vi "例7.4利用XY图显示单条曲线.vi"() -> ()   [LabVIEW 2017]
panel:
  out "XY图 2":cluster{"X":dbl, "Y":dbl}[](graph)
  out "XY图":cluster{dbl[], dbl[]}(graph)
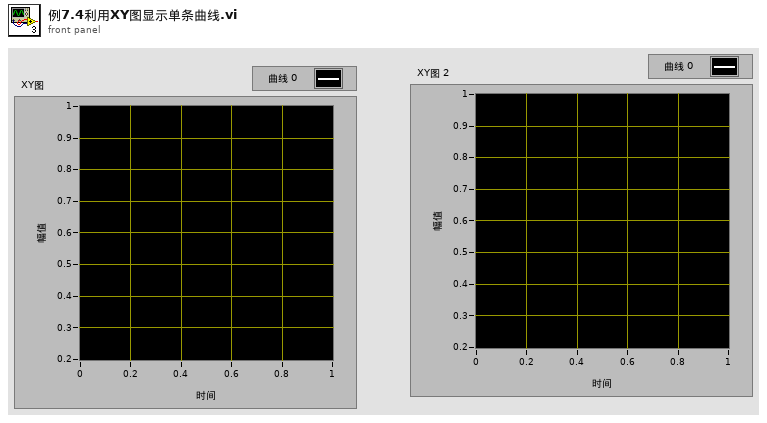
[diagram p1: front panel]
types:
  T1 = cluster{"number: 0 to 1":dbl, "number: 0 to 1":dbl}
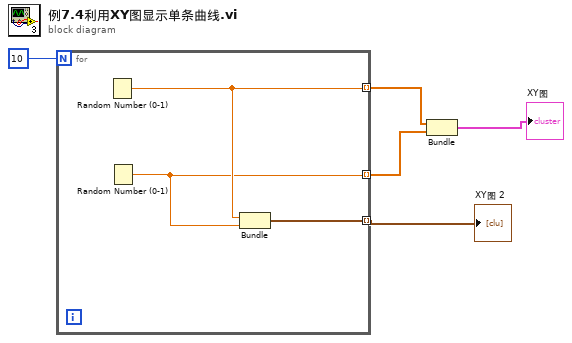
[diagram p0: block diagram]
diagram:
  n1 = for {
    N: 10 -> [_]
    tunnel: [w8] -> w4 mode=indexing
    tunnel: [w7] -> w3 mode=indexing
    tunnel: [w6] -> w1 mode=indexing
    n2 = Random Number (0-1)() -> (number: 0 to 1=w8:dbl)
    n3 = Random Number (0-1)() -> (number: 0 to 1=w7:dbl)
    n4 = Bundle("number: 0 to 1"=w8, "number: 0 to 1"=w7) -> (w6:T1)  [unwired: 1 in]
  }
  "XY图 2" <- w1
  n5 = Bundle(w4, w3) -> (→"XY图":cluster{dbl[], dbl[]})  [unwired: 1 in]
